vi "Pre Launch Init.vi"(11 "ObservingViewable in":refnum<class "ObservingViewable.lvclass">) -> (0 "error out":errorcluster, 3 "ObservingViewable out":refnum<class "ObservingViewable.lvclass">)   [LabVIEW 2017, in "TestPubSubRouting.lvlib" / "ObservingViewable.lvclass"]
doc: "(<B>Filename</B>: Actor Framework.lvlib:Actor.lvclass:Pre Launch Init.vi)\n\nDefines behavior that occurs after the Launch Nested Actor method is invoked but before the actor's Actor Core method begins running.\n\nBy default, this method does nothing. A descendant class may override it to define behavior."
uses:
  ObservingViewable.lvclass
  gpm_packages/@cs/mva-core/Source/IObserver/IObserver/IObserver.lvclass
  gpm_packages/@cs/mva-viewable/Source/IViewable/IViewable/IViewable.lvclass
  C:/Git/mva-framework/Source/Framework/IObserver/IObserver/IObserver.lvclass
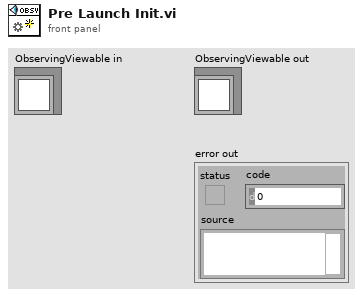
[diagram p1: front panel]
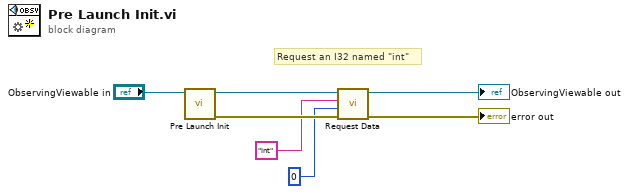
[diagram p0: block diagram]
diagram:
  # "Request an I32 named \"int\""
  n1 = call-parent "Pre Launch Init.vi"("IViewable in"="ObservingViewable in") -> ("error out"=w4:errorcluster, "IViewable out"=w7:refnum<class "ObservingViewable.lvclass">)  [unwired: 9 in]
  n2 = call "Request Data.vi"("error in (no error)"=w4, "Data Type"=0, "Datum Name"="int", "IObserver in"=w7) -> ("error out"=→"error out":errorcluster, "IObserver out"=→"ObservingViewable out":refnum<class "ObservingViewable.lvclass">)  [unwired: 5 in, 1 out]
